vi "Close.vi"(8 "error in (no error)":errorcluster, 11 "navX - I2C in":refnum<class "navX - I2C.lvclass">) -> (0 "error out":errorcluster, 3 "navX - I2C out":refnum<class "navX - I2C.lvclass">)   [LabVIEW 2015, in "navX Library v3.lvlib" / "navX - I2C.lvclass"]
uses:
  navX - I2C.lvclass
  navX - I2C.lvclass/navX - I2C.ctl
  navX - Base/navX - Base.lvclass
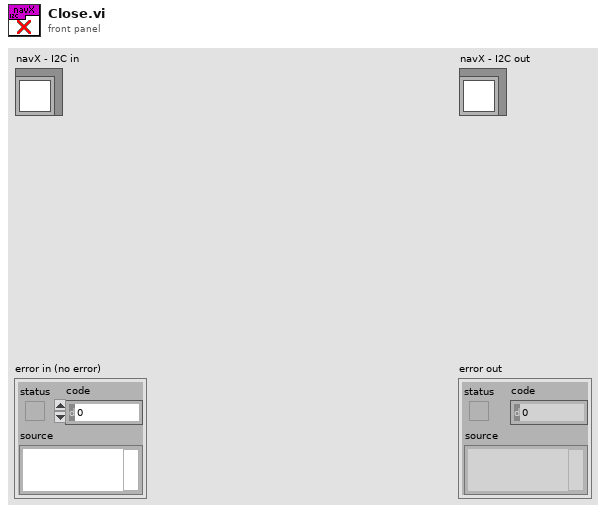
[diagram p1: front panel]
types:
  T1 = typedef "WPI_I2CDevRef.ctl" = cluster{"DevStatus":errorcluster, "Device Address":u8, "Handle":i32, "I2C Bus":T2}
  T2 = typedef "i2c_bus.ctl" = enum16{"I2C On-Board", "I2C MXP", "Invalid"}
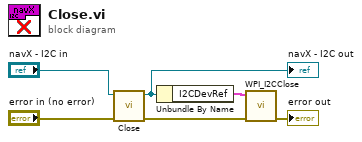
[diagram p0: block diagram]
diagram:
  n1 = call-parent "Close.vi"("error in (no error)"="error in (no error)", "navX - Base in"="navX - I2C in") -> ("error out"=w2:errorcluster, "navX - Base out"=w4:refnum<class "navX - I2C.lvclass">)  [unwired: 8 in]
  "navX - I2C out" <- w4
  n2 = Unbundle By Name(w4) -> ("I2CDevRef"=w3:T1)
  n3 = call <vilib>:"WPI_I2CClose.vi"("error in (no error)"=w2, "I2CDevRef"=w3) -> ("error out"=→"error out":errorcluster)  [unwired: 9 in]
